vi "UnloadAction.vi"(8 "error in (no error)":errorcluster caption="entrée d'erreur (pas d'erreur)", 11 "Tools In":refnum<class "E8267D.lvclass"> caption="DNL_LabVIEW Object in") -> (0 "error out":errorcluster caption="sortie d'erreur", 3 "Tools Out":refnum<class "E8267D.lvclass"> caption="DNL_LabVIEW Object out")   [LabVIEW 2019, in "E8267D.lvclass"]
uses:
  E8267D.lvclass
  C:/Programmes Labview/LabscanV1A/DevicesClass/BaseDevice/BaseDevice.lvclass
  BaseDevice/BaseDevice.lvclass
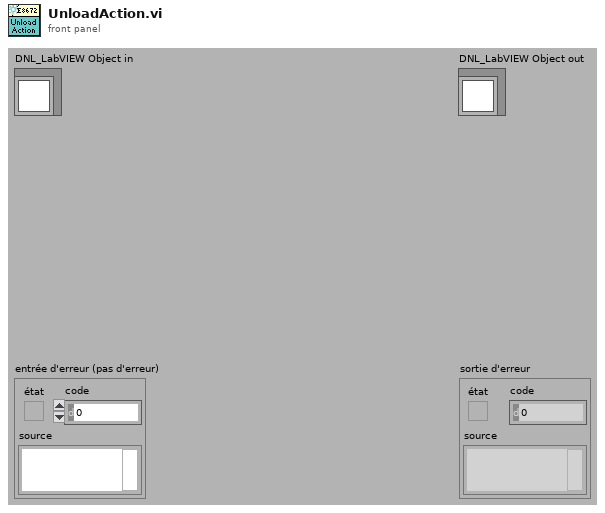
[diagram p1: front panel]
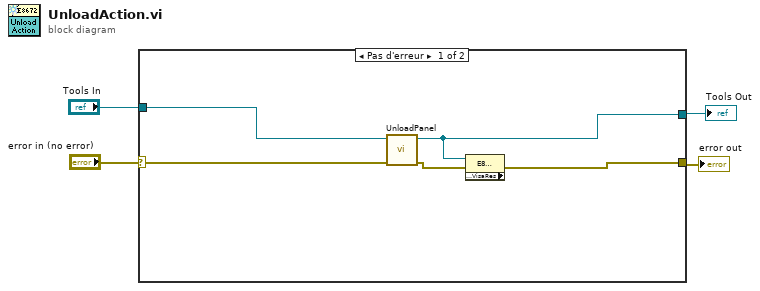
[diagram p0: block diagram]
diagram:
  n1 = case shown="Pas d'erreur" "error in (no error)" {
    selector: "error in (no error)" -> [w9 w10]
    tunnel: [w5 w10] -> w3
    tunnel: [w7 w11] -> w2
    tunnel: "Tools In" -> [w8 w11]
    frame No Error {
      n2 = call "UnloadPanel.vi"("error in (no error)"=w9, "Device en entrée"=w8) -> ("error out"=w6:errorcluster, "Device en sortie"=w7:refnum<class "E8267D.lvclass">)  [unwired: 8 in]
      n3 = property class="E8267D.lvclass" props=["Accessor:VisaRes"](reference=w7, error in=w6) -> (error out=w5:errorcluster)  [unwired: 2 out]
    }
    frame Error {
    }
  }
  "error out" <- w3
  "Tools Out" <- w2
